vi "Convert Tx Rx data to display.vi"(11 "data cluster":T1) -> (3 "Array":string[](array[string]))   [LabVIEW 2020]
uses:
  Data Cluster.ctl
panel:
  # "Send Data:"
  # "Receive Data:"
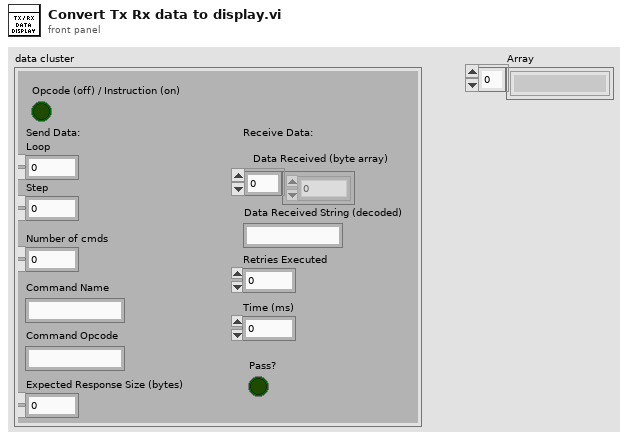
[diagram p1: front panel]
types:
  T1 = typedef "Data Cluster.ctl" = cluster{"Command Name":string, "Command Opcode ":string, "Step":dbl, "Loop":dbl, "Expected Response Size (bytes)":u16, "Number of cmds":dbl, "Data Received (byte array)":u8[], "Retries Executed":u16, "Time (ms)":u16, "Pass?":bool, "Opcode (off) / Instruction (on)":bool, "Data Received String (decoded)":string}
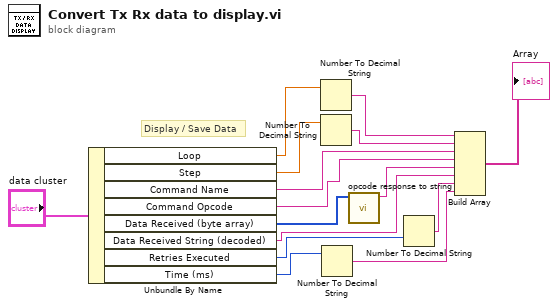
[diagram p0: block diagram]
diagram:
  # "Display / Save Data"
  n1 = Unbundle By Name("data cluster") -> ("Loop"=w6:dbl, "Step"=w7:dbl, "Command Name"=w11:string, "Command Opcode"=w12:string, "Data Received (byte array)"=w13:u8[], "Data Received String (decoded)"=w1:string, "Retries Executed"=w2:u16, "Time (ms)"=w3:u16)
  n2 = Number To Decimal String(number=w6) -> (decimal integer string=w9:string)  [unwired: 1 in]
  n3 = Number To Decimal String(number=w7) -> (decimal integer string=w10:string)  [unwired: 1 in]
  n4 = Number To Decimal String(number=w3) -> (decimal integer string=w5:string)  [unwired: 1 in]
  n5 = call "opcode response to string.vi"("Data Received"=w13) -> ("Response String"=w14:string)  [unwired: 10 in]
  n6 = Number To Decimal String(number=w2) -> (decimal integer string=w4:string)  [unwired: 1 in]
  n7 = Build Array(w9, w10, w11, w12, w14, w1, w4, w5) -> (→"Array":string[])
